vi "Tosca-Wait For Baseline.vi"(0 "Parameters in":refnum<class "Parameters.lvclass">, 11 "error in (no error)":errorcluster) -> (4 "Parameters out":refnum<class "Parameters.lvclass">, 15 "error out":errorcluster)   [LabVIEW 2020]
uses:
  Classes/Parameters/Parameters.lvclass
  Classes/Parameters/Parameters.lvclass/Parameters.ctl
  7dd24b59-b5d2-48ac-a945-9c86996b8694.vi
  Classes/Parameters/Read DAQ.vi
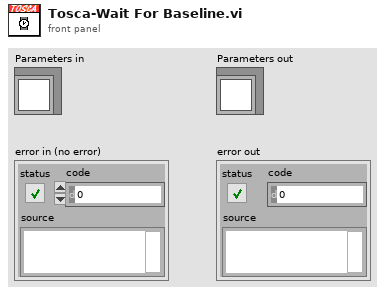
[diagram p1: front panel]
types:
  T1 = typedef "Parameters.lvclass/DAQ.ctl" = cluster{"AO Fs (Hz)":dbl, "DO Fs (Hz)":dbl, "Poll Rate (Hz)":dbl, "Baseline (s)":dbl}
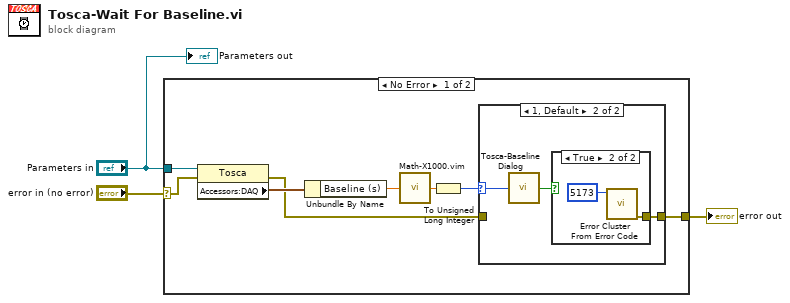
[diagram p0: block diagram]
diagram:
  n1 = case shown="No Error" "error in (no error)" {
    selector: "error in (no error)" -> [w10 w18]
    tunnel: "Parameters in" -> [w11 _]
    tunnel: [w4 w18] -> w2
    frame No Error {
      n2 = property class="Tosca"(reference=w11, error in=w10) -> (error out=w5:errorcluster, "Accessors:DAQ"=w9:T1)  [unwired: 1 out]
      n3 = Unbundle By Name(w9) -> ("Baseline (s)"=w8:dbl)
      n4 = call "Math-X1000.vim"("X"=w8) -> ("1000X"=w7:dbl)
      n5 = To Unsigned Long Integer(number=w7) -> (unsigned 32bit integer=w6:u32)
      n6 = case shown="1, Default" w6 {
        selector: w6 -> [_ w15]
        tunnel: w5 -> [w12 _]
        tunnel: [w12 w13] -> w4
        frame 0 {
        }
        frame 1, Default {
          n7 = call "Tosca-Baseline Dialog.vi"("milliseconds to wait"=w15) -> ("aborted?"=w14:bool)  [unwired: 14 in]
          n8 = case shown="True" w14 {
            tunnel: [_ w16] -> w13
            frame False {
            }
            frame True {
              n9 = call <vilib>:"Error Cluster From Error Code.vi"("error code (0)"=5173) -> ("error out"=w16:errorcluster)  [unwired: 8 in]
            }
          }
        }
      }
    }
    frame Error {
    }
  }
  "error out" <- w2
  "Parameters out" <- "Parameters in"
